vi "check changed.vi"(9 "error in (no error)":errorcluster, 10 "data":variant) -> (1 "error out":errorcluster, 2 "changed?":bool)   [LabVIEW 2017, in "UI-DisplayTable(dev).xctl"]
uses:
  UI-DisplayTable(dev).xctl
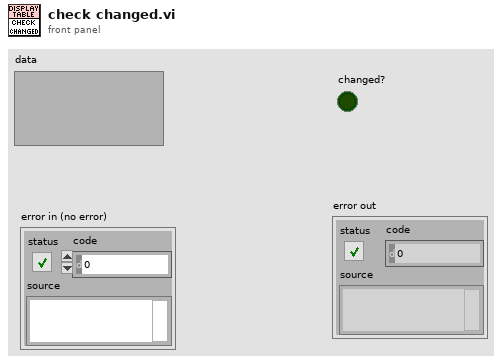
[diagram p1: front panel]
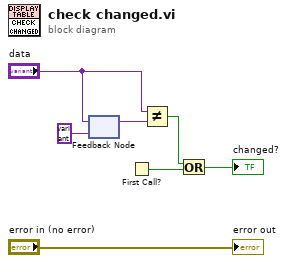
[diagram p0: block diagram]
diagram:
  n1 = feedback-in #1("data") -> ()
  n2 = feedback #1(variant ("data")) -> (w5:variant)
  n3 = First Call?() -> (First Call?: T/F=w3:bool)
  n4 = Not Equal?(x="data", y=w5) -> (x != y?=w2:bool)
  n5 = Or(x=w2, y=w3) -> (x .or. y?=→"changed?":bool)
  "error out" <- "error in (no error)"
